vi "LCDWriteText.vi"(0 "Device In":u64, 1 "Font":u16(ring)=4 items=["FONT_User1"=1, "FONT_User2"=2, "FONT_6x10"=3, "FONT_5x8"=4, "FONT_6x12"=5], 5 "xpos":i32, 7 "ypos":i32, 9 "Text":string, 11 "error in (no error)":errorcluster) -> (4 "Device Out":u64, 15 "error out":errorcluster)   [LabVIEW 2012, in "Phidget LCD.lvlib"]
doc: "${WriteText:Header}"
uses:
  <instrlib>/Phidgets/Phidget LCD/Phidget LCD.lvlib
  <instrlib>/Phidgets/Phidget Common/Phidget Common.lvlib
  phidget22.dll
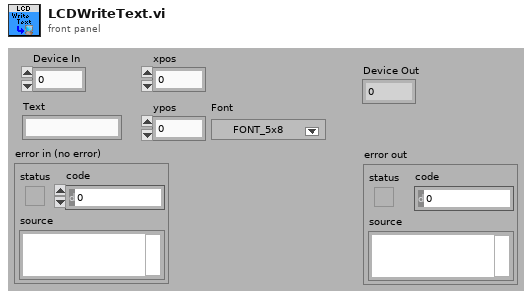
[diagram p1: front panel]
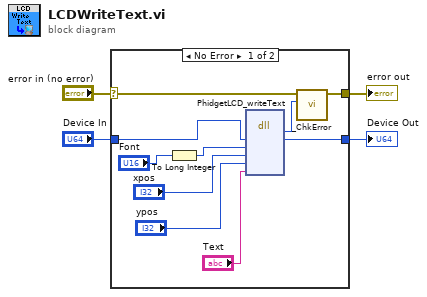
[diagram p0: block diagram]
diagram:
  n1 = case shown="No Error" "error in (no error)" {
    selector: "error in (no error)" -> [w12 w16]
    tunnel: [w11 w16] -> w3
    tunnel: "Device In" -> [w14 w15]
    tunnel: [w13 w15] -> w1
    frame No Error {
      n2 = To Long Integer(number="Font") -> (32bit integer=w8:i32)
      n3 = dll-call lib="phidget22.*" fn="PhidgetLCD_writeText"("phid"=w14, "font"=w8, "xpos"="xpos", "ypos"="ypos", "text"="Text") -> ("return type"=w10:i32, "phid"=w13:u64)  [unwired: 7 in, 2 out]
      n4 = call <instrlib>:"_ChkError.vi"("Return Code"=w10, "error in (no error)"=w12) -> ("error out"=w11:errorcluster)  [unwired: 9 in]
    }
    frame Error {
    }
  }
  "error out" <- w3
  "Device Out" <- w1
